vi "Byte Array to Real Number.vi"(1 "Byte[]":u8[](array[numeric]) format="%.0x") -> (0 "Decimal Number":sgl format="%#.6f")   [LabVIEW 2020, in "Plugin Instrument Driver.lvlib" / "VISA Interface.lvclass"]
doc: "Convers Byte Array into Real Number as per IEEE 754 standard."
uses:
  VISA Interface.lvclass
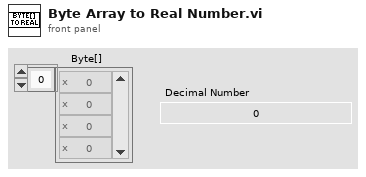
[diagram p1: front panel]
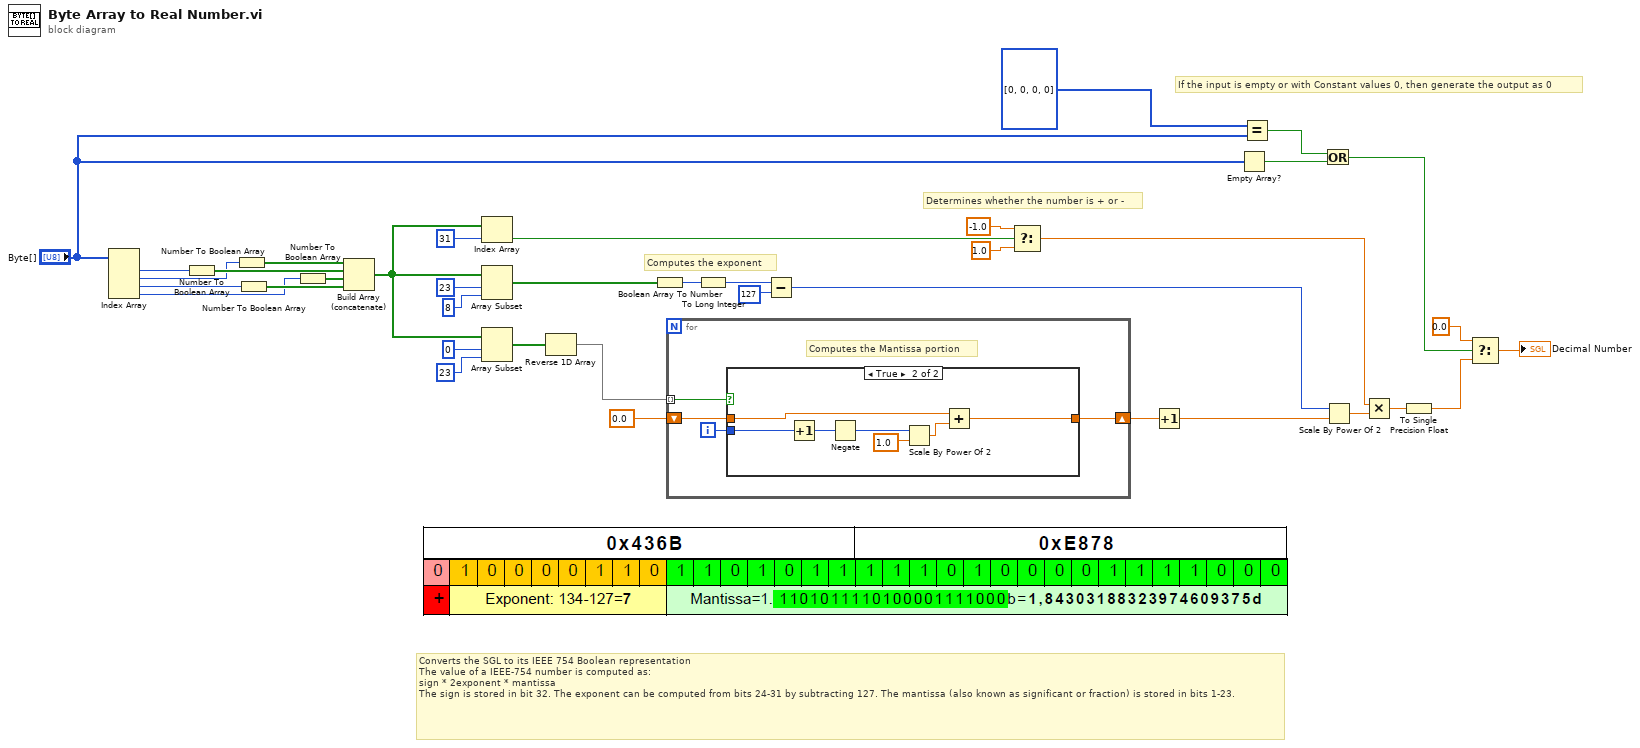
[diagram p0: block diagram]
diagram:
  # "If the input is empty or with Constant values 0, then generate the output as 0"
  # "Computes the exponent"
  # "Determines whether the number is + or -"
  # "Converts the SGL to its IEEE 754 Boolean representation\nThe value of a IEEE-754 number is computed as:\nsign * 2exponent * mantissa\nThe sign is stored in bit 32. The exponent can be computed from bits 24-31 by subtracting 127. The mantissa (also known as significant or fraction) is stored in bits 1-23."
  n1 = Index Array(array="Byte[]") -> (element #1=w24:u8, element #2=w25:u8, element #3=w26:u8, element #4=w27:u8)  [unwired: 4 in]
  n2 = Number To Boolean Array(number=w24) -> (Boolean array=w28:bool[])
  n3 = Number To Boolean Array(number=w25) -> (Boolean array=w29:bool[])
  n4 = Number To Boolean Array(number=w26) -> (Boolean array=w30:bool[])
  n5 = Number To Boolean Array(number=w27) -> (Boolean array=w31:bool[])
  n6 = Build Array (concatenate)(w29, w28, w31, w30) -> (w32:bool[])
  n7 = Index Array(array=w32, index=31) -> (element=w13:bool)
  n8 = Array Subset(array=w32, index=23, length=8) -> (w9:bool[])
  n9 = Array Subset(array=w32, index=0, length=23) -> (w38:bool[])
  n10 = Reverse 1D Array(array=w38) -> (reversed array=w14:bool[])
  n11 = Boolean Array To Number(Boolean array=w9) -> (number=w22:u32)
  n12 = for {
    tunnel: w14 -> [w42] mode=indexing
    shift-right: [w39] -> w18
    shift-left: 0.0 -> [w40]
    i -> [w41]
    # "Computes the Mantissa portion"
    n13 = case shown="True" w42 {
      tunnel: w41 -> [_ w50]
      tunnel: w40 -> [w43 w46]
      tunnel: [w43 w44] -> w39
      frame False {
      }
      frame True {
        n14 = Increment(x=w50) -> (x+1=w49:i32)
        n15 = Negate(x=w49) -> (-x=w48:i32)
        n16 = Scale By Power Of 2(n=w48, x=1.0) -> (x*2^n=w45:dbl)
        n17 = Add(x=w46, y=w45) -> (x+y=w44:dbl)
      }
    }
  }
  n18 = To Long Integer(number=w22) -> (32bit integer=w23:i32)
  n19 = Subtract(x=w23, y=127) -> (x-y=w15:i32)
  n20 = Select(t=-1.0, s=w13, f=1.0) -> (s? t:f=w10:dbl)
  n21 = Increment(x=w18) -> (x+1=w16:dbl)
  n22 = Empty Array?(array="Byte[]") -> (empty?=w3:bool)
  n23 = Equal?(x=u8[] [0, 0, 0, 0], y="Byte[]") -> (x = y?=w2:bool)
  n24 = Or(x=w2, y=w3) -> (x .or. y?=w1:bool)
  n25 = Scale By Power Of 2(n=w15, x=w16) -> (x*2^n=w20:dbl)
  n26 = Multiply(x=w10, y=w20) -> (x*y=w21:dbl)
  n27 = To Single Precision Float(number=w21) -> (single precision float=w8:sgl)
  n28 = Select(t=sgl 0.0, s=w1, f=w8) -> (s? t:f=→"Decimal Number":sgl)
